vi "my글로벌.vi"() -> ()   [LabVIEW 2014]
panel:
  out "Stop":bool
  in  "Data":dbl
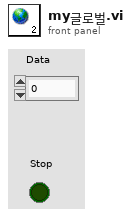
[diagram p1: front panel]
diagram:
